vi "26_Generating nos using array.vi"() -> ()   [LabVIEW 2018]
panel:
  out "Maximum":dbl
  out "Minimum":dbl
  out "Array":dbl[](array[numeric])
  # "WAP to generate 5 numbers and store in array"
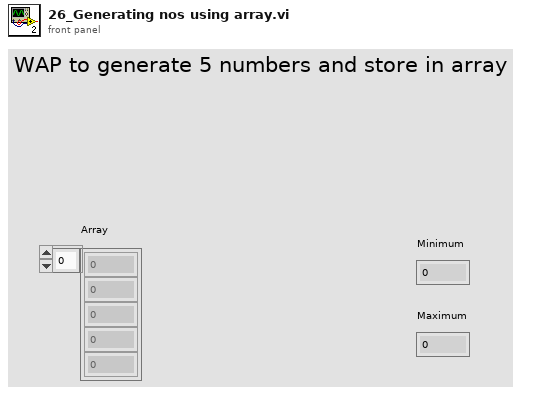
[diagram p1: front panel]
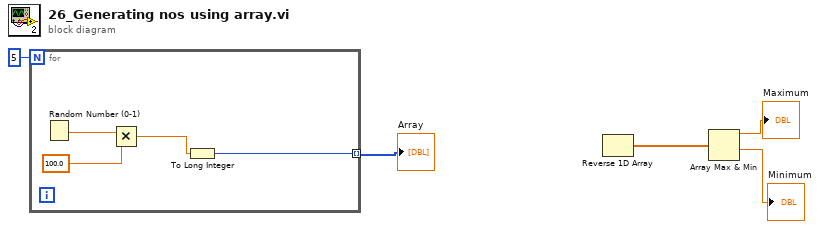
[diagram p0: block diagram]
diagram:
  n1 = for {
    N: 5 -> [_]
    tunnel: [w7] -> w4 mode=indexing
    n2 = Random Number (0-1)() -> (number: 0 to 1=w9:dbl)
    n3 = Multiply(x=w9, y=100.0 ("x")) -> (x*y=w8:dbl)
    n4 = To Long Integer(number=w8) -> (32bit integer=w7:i32)
  }
  "Array" <- w4
  n5 = Reverse 1D Array() -> (reversed array=w3:dbl[])  [unwired: 1 in]
  n6 = Array Max & Min(array=w3) -> (max value=→"Maximum":dbl, min value=→"Minimum":dbl)  [unwired: 2 out]
